vi "Write Table of Content.vi"(0 "PDF Report IN":refnum<class "PDF Report Class.lvclass">=refnum, 11 "error in (no error)":errorcluster) -> (4 "PDF Report OUT":refnum<class "PDF Report Class.lvclass">, 8 "TOC page":cluster{"Start":i32, "Number":i32}, 15 "error out":errorcluster)   [LabVIEW 2020, in "Exaprom PDF.lvlib"]
doc: "Version 1.12.0\nDeveloped by Jean-Marc Simard\nCopyright © 2013, Exaprom Inc.\nAll rights reserved.\nLicense: BSD\n\nWith iTextSharp 4.1.6 (http://itextsharp.sourceforge.net)\nunder Mozilla Public License Version 1.1\n(http://www.mozilla.org/MPL/MPL-1.1.html)"
uses:
  <userlib>/labview-PDF-writer-master/Exaprom PDF.lvlib
  <userlib>/labview-PDF-writer-master/LV Class/PDF Report Class/PDF Report Class.lvclass
  <userlib>/labview-PDF-writer-master/LV Class/Fonts Class/Font Class.lvclass
  <userlib>/labview-PDF-writer-master/LV Class/Header and Footer Class/Header and Footer Class.lvclass
  <userlib>/labview-PDF-writer-master/Controls/Initialization Controls/Defaut Paragraphe and Line Spacing.ctl
  <userlib>/labview-PDF-writer-master/Controls/Text Controls/Texte alignement.ctl
  <userlib>/labview-PDF-writer-master/Controls/Text Controls/Line spacing.ctl
  C:/Program Files (x86)/National Instruments/LabVIEW 2020/user.lib/labview-PDF-writer-master/DLL/itextsharp.dll
  DLL/itextsharp.dll
  <userlib>/labview-PDF-writer-master/Controls/Font Controls/Font size.ctl
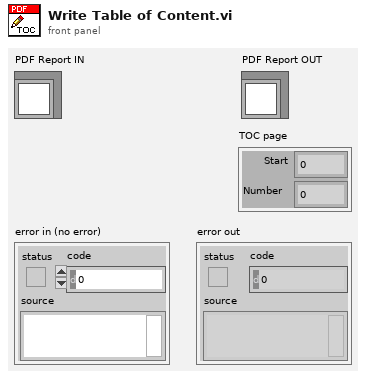
[diagram p1: front panel]
types:
  T1 = typedef "Exaprom PDF.lvlib/Defaut Paragraphe and Line Spacing.ctl" = cluster{" Aligment":T2, "Line spacing":T3}
  T2 = typedef "Exaprom PDF.lvlib/Texte alignement.ctl" = enum16{"Select", "CENTER", "JUSTIFY", "LEFT", "RIGHT"}
  T3 = typedef "Exaprom PDF.lvlib/Line spacing.ctl" = enum16{"Select", "1.0", "1.5", "2.0"}
  T4 = typedef "Exaprom PDF.lvlib/Font size.ctl" = sgl
  T5 = typedef "Exaprom PDF.lvlib/TOC.ctl" = cluster{"Title":string, "Title Font":T6, "Chapter and section Font":T6, "First TOC page":u16, "Add TOC?":bool}
  T6 = typedef "Exaprom PDF.lvlib/Font complete cluster.ctl" = cluster{"Name":string, "Size":T4, "Color":T7, "Style":cluster{"Bold":bool, "Italic":bool, "Underline":bool, "Strikeout":bool}, "Type":T8}
  T7 = typedef "Exaprom PDF.lvlib/Font color.ctl" = u32
  T8 = typedef "Exaprom PDF.lvlib/Type and encoding.ctl" = cluster{"Type&direction":T9, "Embedded":bool, "Encoding":string}
  T9 = typedef "Exaprom PDF.lvlib/Type and run direction.ctl" = enum16{"Select", "ASCII", "UTF-16", "UTF-16 (default)", "UTF-16 (LTR)", "UTF-16 (RTL)"}
  T10 = typedef "Exaprom PDF.lvlib/TOC Line.ctl" = cluster{"Title":string, "Level":u16, "GoTo Page":u16, "GoTo Position":u16, "Destination":string, "Type & run direction":T9}
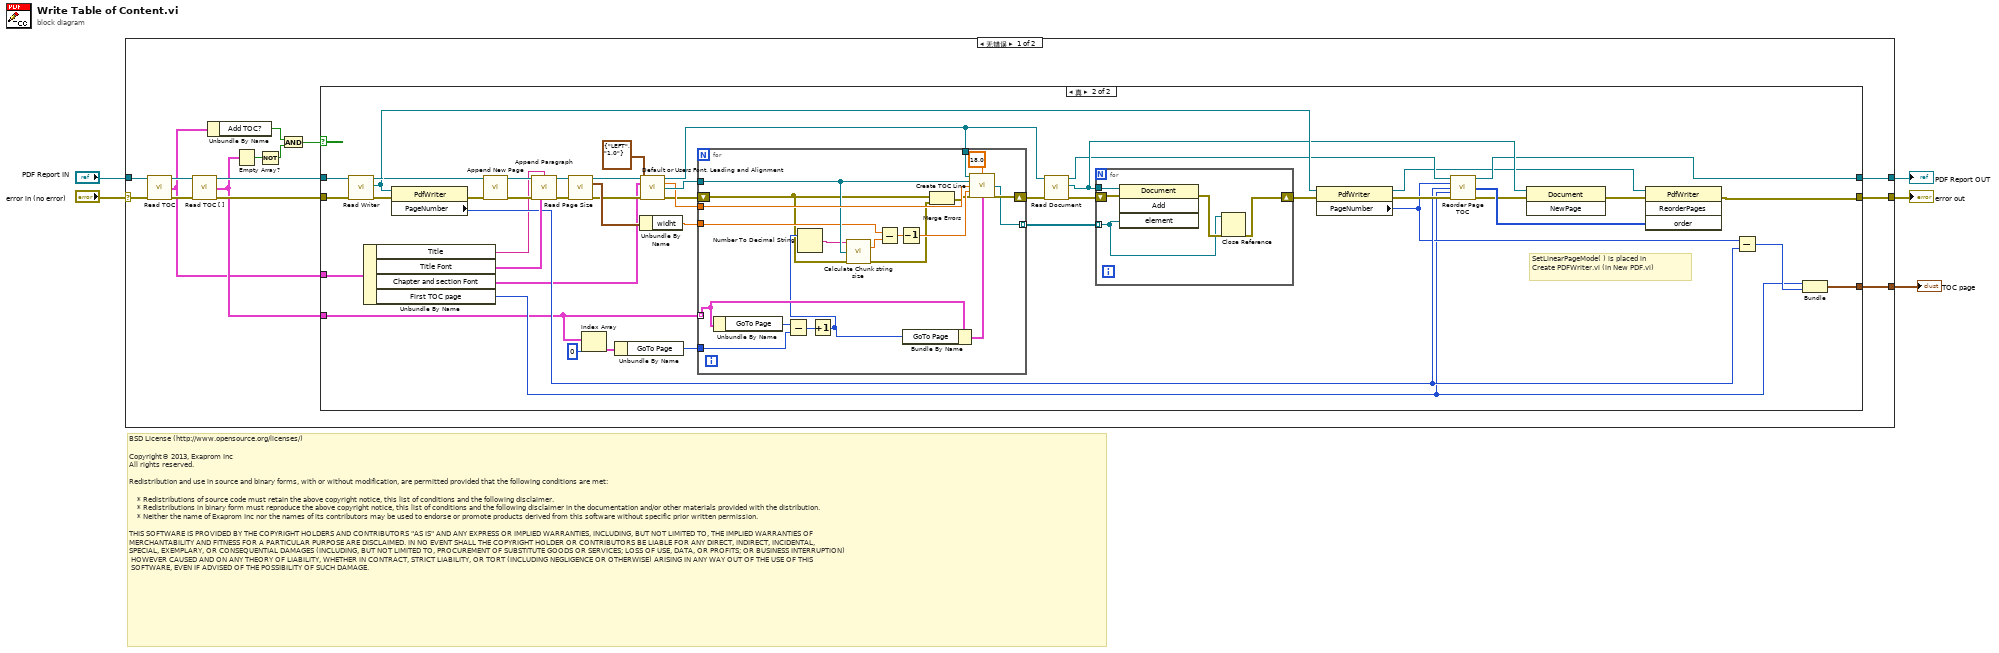
[diagram p0: block diagram]
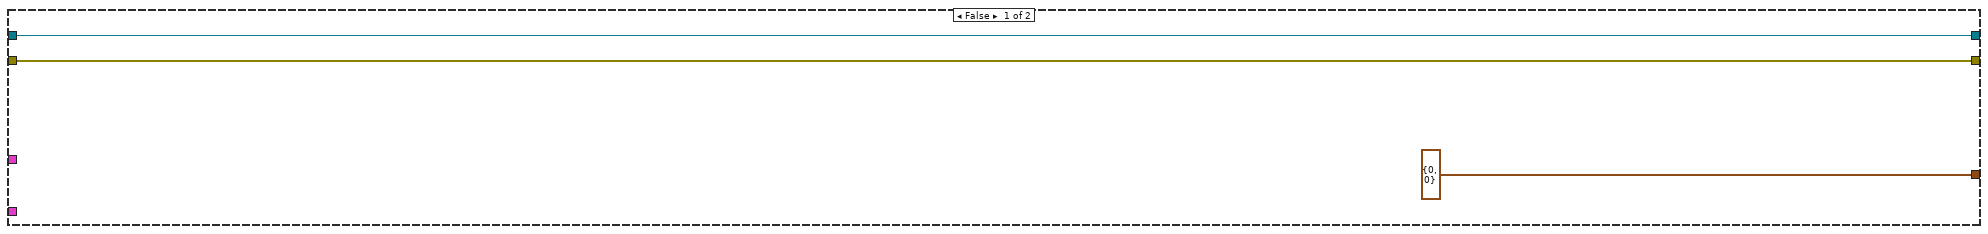
[diagram p2: hidden frame]
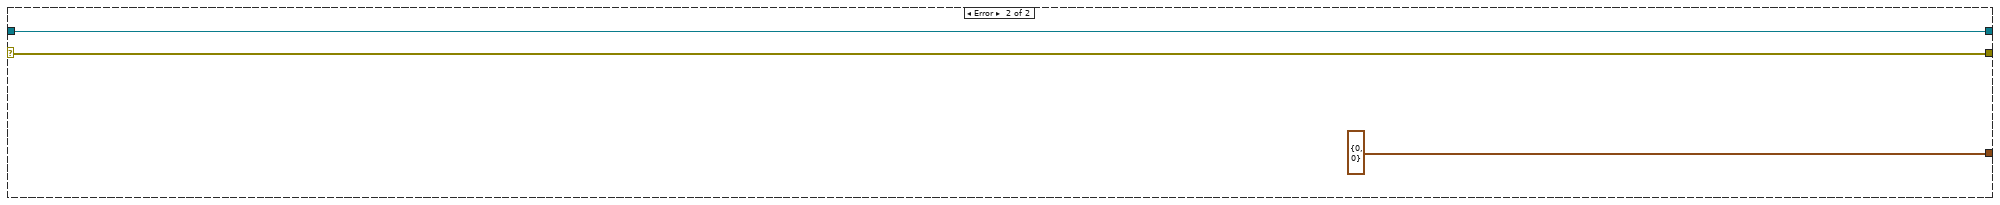
[diagram p3: hidden frame]
diagram:
  # "BSD License (http://www.opensource.org/licenses/)\n\nCopyright© 2013, Exaprom Inc\nAll rights reserved.\n\nRedistribution and use in source and binary forms, with or without modification, are permitted provided that the following conditions are met:\n\n    * Redistributions of source code must retain the above copyright notice, this list of conditions and the following disclaimer.\n    * Redistributions in binary form must reproduce the above copyright notice, this list of conditions and the following disclaimer in the documentation and/or other materials provided with the distribution.\n    * Neither the name of Exaprom Inc nor the names of its contributors may be used to endorse or promote products derived from this software without specific prior written permission.\n\nTHIS SOFTWARE IS PROVIDED BY THE COPYRIGHT HOLDERS AND CONTRIBUTORS \"AS IS\" AND ANY EXPRESS OR IMPLIED WARRANTIES, INCLUDING, BUT NOT LIMITED TO, THE IMPLIED WARRANTIES OF \nMERCHANTABILITY AND FITNESS FOR A PARTICULAR PURPOSE ARE DISCLAIMED. IN NO EVENT SHALL THE COPYRIGHT HOLDER OR CONTRIBUTORS BE LIABLE FOR ANY DIRECT, INDIRECT, INCIDENTAL,\nSPECIAL, EXEMPLARY, OR CONSEQUENTIAL DAMAGES (INCLUDING, BUT NOT LIMITED TO, PROCUREMENT OF SUBSTITUTE GOODS OR SERVICES; LOSS OF USE, DATA, OR PROFITS; OR BUSINESS INTERRUPTION)\n HOWEVER CAUSED AND ON ANY THEORY OF LIABILITY, WHETHER IN CONTRACT, STRICT LIABILITY, OR TORT (INCLUDING NEGLIGENCE OR OTHERWISE) ARISING IN ANY WAY OUT OF THE USE OF THIS\n SOFTWARE, EVEN IF ADVISED OF THE POSSIBILITY OF SUCH DAMAGE."
  n1 = case shown="无错误" "error in (no error)" {
    selector: "error in (no error)" -> [w7 w95]
    tunnel: "PDF Report IN" -> [w8 w96]
    tunnel: [w20 w96] -> w4
    tunnel: [w19 w95] -> w3
    tunnel: [w6 cluster{"PageNumber":i32, i32} {"PageNumber"=0, 0}] -> w1
    frame No Error {
      n2 = call-dynamic "Read TOC.vi"("PDF Report Class in"=w8, "error in (no error)"=w7) -> ("PDF Report Class out"=w15:refnum<class "PDF Report Class.lvclass">, "TOC"=w9:T5, "error out"=w14:errorcluster)  [unwired: 11 in]
      n3 = call-dynamic "Read TOC [ ].vi"("PDF Report Class in"=w15, "error in (no error)"=w14) -> ("PDF Report Class out"=w18:refnum<class "PDF Report Class.lvclass">, "TOC [ ]"=w16:T10[], "error out"=w17:errorcluster)  [unwired: 11 in]
      n4 = Unbundle By Name(w9) -> ("Add TOC?"=w11:bool)
      n5 = Empty Array?(array=w16) -> (empty?=w13:bool)
      n6 = Not(x=w13) -> (.not. x?=w12:bool)
      n7 = And(x=w11, y=w12) -> (x .and. y?=w10:bool)
      n8 = case shown="真" w10 {
        tunnel: [w23 w41] -> w20
        tunnel: [w22 w37] -> w19
        tunnel: w18 -> [w23 w60]
        tunnel: w17 -> [w22 w57]
        tunnel: w16 -> [_ w30]
        tunnel: w9 -> [_ w51]
        tunnel: [cluster{"PageNumber":i32, i32} {"PageNumber"=0, 0} w34] -> w6
        frame False {
        }
        frame True {
          # "SetLinearPageMode( ) is placed in\nCreate PDFWriter.vi (in New PDF.vi)"
          n9 = call-dynamic "Read Writer.vi"("error in (no error)"=w57, "PDF Report Class in"=w60) -> ("error out"=w56:errorcluster, "Writer"=w46:refnum<k24>, "PDF Report Class out"=w58:refnum<class "PDF Report Class.lvclass">)  [unwired: 7 in]
          n10 = Unbundle By Name(w51) -> ("Title"=w25:string, "Title Font"=w49:T6, "Chapter and section Font"=w24:T6, "First TOC page"=w31:u16)
          n11 = property class="PdfWriter"(reference=w46, error in=w56) -> (error out=w55:errorcluster, "PageNumber"=w38:i32)  [unwired: 1 out]
          n12 = call <userlib>:"Append New Page.vi"("PDF Report"=w58, "error in (no error)"=w55) -> ("PDF Report duplicate"=w59:refnum<class "PDF Report Class.lvclass">, "error OUT"=w53:errorcluster)  [unwired: 12 in]
          n13 = call <userlib>:"Append Paragraph.vi"("PDF Report"=w59, "Text"=w25, "error in (no error)"=w53, "Font"=w49) -> ("PDF Report duplicate"=w54:refnum<class "PDF Report Class.lvclass">, "error out"=w52:errorcluster)  [unwired: 10 in]
          n14 = call <userlib>:"Read Page Size.vi"("PDF Report"=w54, "error in (no error)"=w52) -> ("PDF Report duplicate"=w32:refnum<class "PDF Report Class.lvclass">, "Text zone (points)"=w62:cluster{"widht":sgl, "height":sgl}, "error out"=w33:errorcluster)  [unwired: 10 in, 1 out]
          n15 = Index Array(array=w30, index=0) -> (element=w29:T10)
          n16 = Unbundle By Name(w29) -> ("GoTo Page"=w27:u16)
          n17 = Unbundle By Name(w62) -> ("widht"=w61:sgl)
          n18 = call <userlib>:"Default or Users Font, Leading and Alignment.vi"("PDF Report"=w32, "Font"=w24, "Paragraphe cluster"=T1 {" Aligment"=enum."LEFT", "Line spacing"=enum."1.0"}, "error in (no error)"=w33) -> ("PDF Report duplicate"=w26:refnum<class "PDF Report Class.lvclass">, "Leading"=w67:T4, "Font Ref"=w68:refnum<k24>, "error out"=w66:errorcluster)  [unwired: 5 in, 3 out]
          n19 = for {
            tunnel: w30 -> [w81] mode=indexing
            tunnel: w68 -> [w90]
            tunnel: w67 -> [w92]
            tunnel: w61 -> [w88]
            tunnel: [w91] -> w64 mode=indexing
            shift-right: [w93] -> w65
            shift-left: w66 -> [w75]
            tunnel: w27 -> [w83]
            tunnel: w26 -> [w74]
            n20 = Unbundle By Name(w81) -> ("GoTo Page"=w84:u16)
            n21 = Subtract(x=w84, y=w83) -> (x-y=w82:u16)
            n22 = Increment(x=w82) -> (x+1=w80:u16)
            n23 = Number To Decimal String(number=w80) -> (decimal integer string=w78:string)  [unwired: 1 in]
            n24 = call <userlib>:"Calculate Chunk string size.vi"("String"=w78, "Font refnum"=w90, "error in (no error)"=w75) -> ("Width"=w89:sgl, "error out"=w76:errorcluster)  [unwired: 9 in, 2 out]
            n25 = Subtract(x=w88, y=w89) -> (x-y=w87:sgl)
            n26 = Decrement(x=w87) -> (x-1=w86:sgl)
            n27 = Bundle By Name(cluster=w81, "GoTo Page"=w80) -> (w79:T10)
            n28 = Merge Errors(w75, w76) -> (w77:errorcluster)
            n29 = call <userlib>:"Create TOC Line.vi"("PDF Report IN"=w74, "Indentation (points)"=T4 18.0, "Font Ref"=w90, "Font Size"=w92, "Width (points)"=w86, "error in (no error)"=w77, "TOC Line"=w79) -> ("Paragraph"=w91:refnum<k24>, "error out"=w93:errorcluster)  [unwired: 6 in, 1 out]
          }
          n30 = call-dynamic "Read Document.vi"("error in (no error)"=w65, "PDF Report Class in"=w26) -> ("error out"=w63:errorcluster, "Document"=w45:refnum<k24>, "PDF Report Class out"=w43:refnum<class "PDF Report Class.lvclass">)  [unwired: 7 in]
          n31 = for {
            tunnel: w64 -> [w70] mode=indexing
            shift-right: [w69] -> w48
            shift-left: w63 -> [w73]
            tunnel: w45 -> [w72]
            n32 = invoke class="Document" method="Add"(reference=w72, error in=w73, "element"=w70) -> (error out=w71:errorcluster)  [unwired: 1 in, 3 out]
            n33 = Close Reference(reference=w70, error in (no error)=w71) -> (error out=w69:errorcluster)
          }
          n34 = property class="PdfWriter"(reference=w46, error in=w48) -> (reference out=w39:refnum<k24>, error out=w44:errorcluster, "PageNumber"=w36:i32)
          n35 = call <userlib>:"Reorder Page TOC.vi"("PDF Report IN"=w43, "Number pages after TOC"=w36, "Number pages before TOC"=w38, "TOC start at page"=w31, "error in (no error)"=w44) -> ("PDF Report OUT"=w41:refnum<class "PDF Report Class.lvclass">, "Pages [ ]"=w42:i32[], "error out"=w40:errorcluster)  [unwired: 8 in]
          n36 = invoke class="Document" method="NewPage"(reference=w45, error in=w40) -> (error out=w47:errorcluster)  [unwired: 1 in, 2 out]
          n37 = invoke class="PdfWriter" method="ReorderPages"(reference=w39, error in=w47, "order"=w42) -> (error out=w37:errorcluster)  [unwired: 1 in, 3 out]
          n38 = Subtract(x=w36, y=w38) -> (x-y=w35:i32)
          n39 = Bundle("First TOC page"=w31, w35) -> (w34:cluster{"First TOC page":u16, i32})  [unwired: 1 in]
        }
      }
    }
    frame Error {
    }
  }
  "PDF Report OUT" <- w4
  "error out" <- w3
  "TOC page" <- w1
